vi "ValueTable_head1.vi"(2 "error in 2":errorcluster, 3 "Файл записи":refnum<file>, 6 "Количество датчиков":i32, 7 "Cluster":T1) -> (0 "error out":errorcluster, 1 "Файл записи 2":refnum<file>)   [LabVIEW 2018]
doc: "Доавляет в шапку таблицы txt-файла названия измеряемой величины и её единицы измерения"
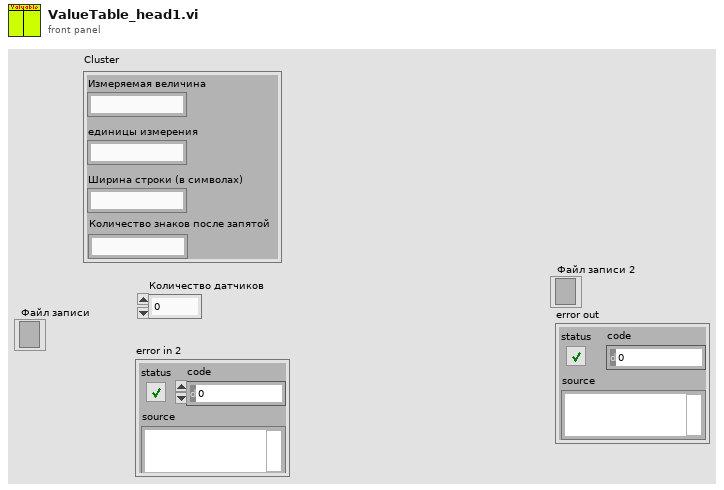
[diagram p1: front panel]
types:
  T1 = cluster{"Измеряемая величина":string, "единицы измерения":string, "Ширина строки (в символах)":string, "Количество знаков после запятой":string}
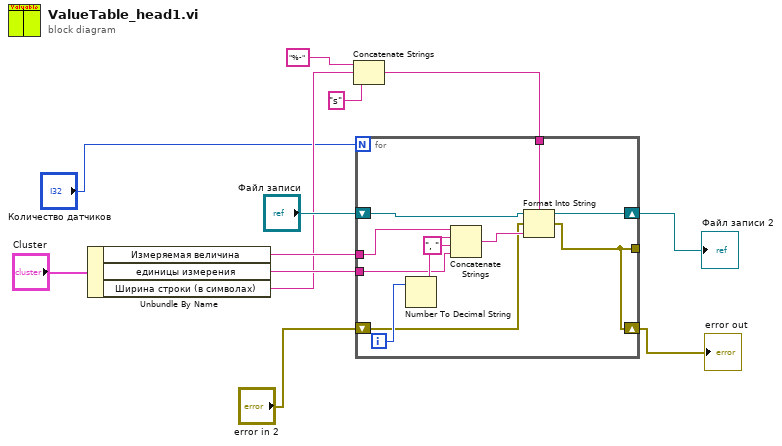
[diagram p0: block diagram]
diagram:
  n1 = Unbundle By Name("Cluster") -> ("Измеряемая величина"=w4:string, "единицы измерения"=w3:string, "Ширина строки (в символах)"=w2:string)
  n2 = Concatenate Strings("%-" ("string"), w2, "s" ("string")) -> (w6:string)
  n3 = for {
    N: "Количество датчиков" -> [_]
    shift-right: [w19] -> w11
    shift-left: "Файл записи" -> [w20]
    shift-right: [w16] -> w9
    shift-left: "error in 2" -> [w17]
    tunnel: [w16] -> _
    tunnel: w6 -> [w15]
    tunnel: w4 -> [w14]
    tunnel: w3 -> [w13]
    i -> [w22]
    n4 = Number To Decimal String(number=w22) -> (decimal integer string=w23:string)  [unwired: 1 in]
    n5 = Concatenate Strings(w14, w23, ", " ("string"), w13) -> (w21:string)
    n6 = Format Into String(format string=w15, initial string=w20, error in=w17, w21) -> (resulting string=w19:refnum<file>, error out=w16:errorcluster)
  }
  "Файл записи 2" <- w11
  "error out" <- w9
